vi "Scope AP Meas test.vi"() -> ()   [LabVIEW 2018]
uses:
  SPD Stand/typedefs/SPD.Stand Ctrl.ctl
  Instruments/SPD HID Interface/hidSPDLibForLabView/LibVIs/hidSPD Controls/hidSPD Device Session.ctl
  Instruments/SPD HID Interface/hidSPDLibForLabView/LibVIs/hidSPD Controls/hidSPD Controller.ctl
  Instruments/SPD HID Interface/hidSPDLibForLabView/LibVIs/hidSPD Controls/hidSPD SPD Type.ctl
  Instruments/KC705 DevBoard/typedefs/DevB.Session.ctl
  Instruments/KeySight 53230A/typedefs/FreqC.Session.ctl
  Instruments/KeySight 8164B/KeySight 8164B LAN InstrLib/typedefs/KeySight 8164B control.ctl
  Instruments/LeCroy SDA830/typedefs/LeCroy.Session.ctl
  SPD Stand/typedefs/SPD.Events.ctl
  SPD Stand/ConfigFile/SPD.Config File ctrl.ctl
  <vilib>/Utility/config.llb/Config Data RefNum.ctl
  SPD Stand/typedefs/SPD.Meas Result.ctl
  SPD Stand/typedefs/SPD.Queues.ctl
  SPD Stand/typedefs/SPD.Stand state.ctl
  Instruments/SPD HID Interface/hidSPDLibForLabView/hidSPDLibForLabView.lvlib
  Instruments/KeySight 8164B/KeySight 8164B LAN InstrLib.lvlib
  <vilib>/Utility/config.llb/NI_LVConfig.lvlib
panel:
  out "Histo":dbl[](graph)
  out "Error Out":errorcluster
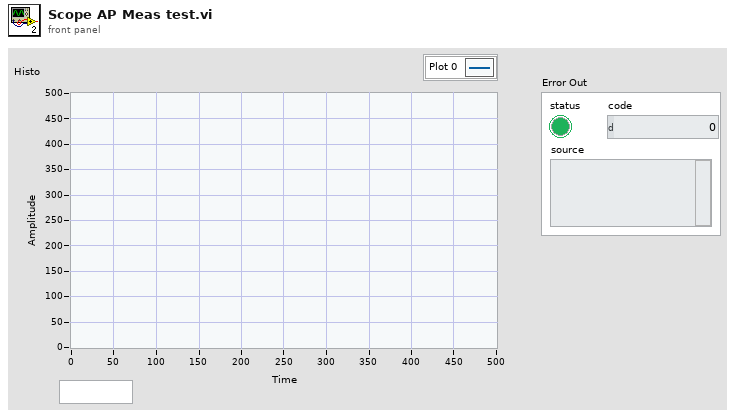
[diagram p1: front panel]
types:
  T1 = typedef "SPD.Stand Ctrl.ctl" = cluster{"spdDeviceSession":T2, "DevBSession":T5, "FreqCSession":T6, "8164BSession":T7, "LeCroySession":T8, "Events":T9, "configFile":T10, "SPD.Result":T12, "SPD.Queues":T13, "Console":refnum<vi>}
  T2 = typedef "hidSPDLibForLabView.lvlib/hidSPD Device Session.ctl" = cluster{"spdRef":u64, "connected":bool, "spdName":string, "hidSPD.Controller":T3, "hidSPD.Sturtup Values":T3, "SPD Type":T4}
  T3 = typedef "hidSPDLibForLabView.lvlib/hidSPD Controller.ctl" = cluster{"TSet":sgl, "HV_bias":sgl, "DDS_stb_code":u16}
  T4 = typedef "hidSPDLibForLabView.lvlib/hidSPD SPD Type.ctl" = enum16{"Free Run", "Strobe"}
  T5 = typedef "DevB.Session.ctl" = cluster{"DevBRef":refnum<visa-resource-name>, "connected":bool}
  T6 = typedef "FreqC.Session.ctl" = cluster{"FreqCRef":refnum<visa-resource-name>, "timeout":dbl, "Gate":dbl, "connected":bool}
  T7 = typedef "KeySight 8164B LAN InstrLib.lvlib/KeySight 8164B control.ctl" = cluster{"Connection ID":refnum<k5>, "Connected":bool, "Info":string, "Slots Info":string[]}
  T8 = typedef "LeCroy.Session.ctl" = cluster{"LeCroySession":refnum<visa-resource-name>, "connected":bool}
  T9 = typedef "SPD.Events.ctl" = cluster{"DCRTest":refnum<user-event>, "Stop":refnum<user-event>}
  T10 = typedef "SPD.Config File ctrl.ctl" = cluster{"configFile ref":T11, "configFile path":path}
  T11 = typedef "NI_LVConfig.lvlib/Config Data RefNum.ctl" = refnum<k1>
  T12 = typedef "SPD.Meas Result.ctl" = cluster{"HV_Bias":dbl[][][], "Stb_code":dbl[], "Temprature":dbl[], "Data":dbl[][][][], "DateTime":string}
  T13 = typedef "SPD.Queues.ctl" = cluster{"state queue":refnum<queue>}
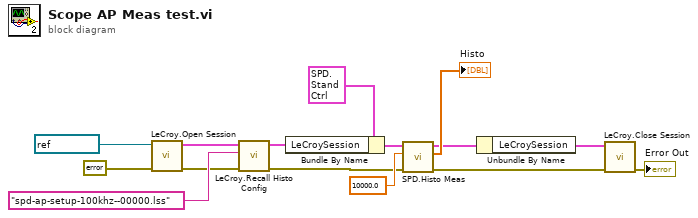
[diagram p0: block diagram]
diagram:
  n1 = call "LeCroy.Open Session.vi"("Error In"=errorcluster {"status"=FALSE, "code"=0, "source"=""}, "VISA resource name"=refnum<visa-resource-name> "LeCroy") -> ("Error Out"=w7:errorcluster, "LeCroy.Session out"=w9:T8)  [unwired: 8 in]
  n2 = call "LeCroy.Recall Histo Config.vi"("Error In"=w7, "Filename (panel.lss)"="spd-ap-setup-100khz--00000.lss", "LeCroy.Session in"=w9) -> ("Error Out"=w3:errorcluster, "LeCroy.Session out"=w6:T8)  [unwired: 7 in]
  n3 = Bundle By Name(cluster=T1 {"spdDeviceSession"={"spdRef"=0, "connected"=FALSE, "spdName"="", "hidSPD.Controller"={"TSet"=0.0, "HV_bias"=0.0, "DDS_stb_code"=0}, "hidSPD.Sturtup Values"={"TSet"=0.0, "HV_bias"=0.0, "DDS_stb_code"=0}, "SPD Type"=enum."Free Run"}, "DevBSession"={"DevBRef"="", "connected"=FALSE}, "FreqCSession"={"FreqCRef"="", "timeout"=0.0, "Gate"=0.0, "connected"=FALSE}, "8164BSession"={"Connection ID"=refnum, "Connected"=FALSE, "Info"="", "Slots Info"=[]}, "LeCroySession"={"LeCroySession"="", "connected"=FALSE}, "Events"={"DCRTest"=refnum, "Stop"=refnum}, "configFile"={"configFile ref"=refnum, "configFile path"=path ""}, "SPD.Result"={"HV_Bias"=[], "Stb_code"=[], "Temprature"=[], "Data"=[], "DateTime"=""}, "SPD.Queues"={"state queue"=refnum}, "Console"=refnum} ("SPD.Stand Ctrl in"), "LeCroySession"=w6) -> (w4:T1)
  n4 = call "SPD.Histo Meas.vi"("Error In"=w3, "Histo length"=10000.0, "SPD.Stand Ctrl in"=w4) -> ("Error Out"=w12:errorcluster, "AP Histo"=→"Histo":dbl[], "SPD.Stand Ctrl out"=w2:T1)  [unwired: 6 in]
  n5 = Unbundle By Name(w2) -> ("LeCroySession"=w1:T8)
  n6 = call "LeCroy.Close Session.vi"("Error In"=w12, "LeCroy.Session in"=w1) -> ("Error Out"=→"Error Out":errorcluster)  [unwired: 9 in]
